vi "Write Both Fan States.vi"(8 "error in (no error)":errorcluster, 9 "Fan B State":bool, 10 "Fan A State":bool, 11 "Dual Fan in":refnum<class "Dual Fan.lvclass">) -> (0 "error out":errorcluster)   [LabVIEW 2018, in "Dual Fan.lvlib" / "Dual Fan.lvclass"]
doc: "Child classes should override this method to set the fan states. True means to turn the fan on, false means to turn the fan off. This method is NOT guaranteed to only be called on state transitions -- the fans may already be in the given state."
uses:
  Dual Fan.lvclass
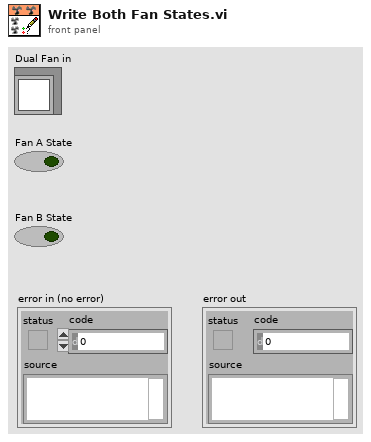
[diagram p1: front panel]
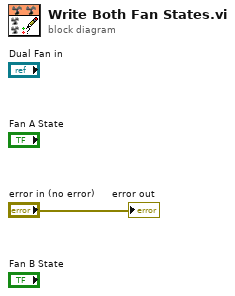
[diagram p0: block diagram]
diagram:
  "error out" <- "error in (no error)"
